vi "ax position control test constant.vi"() -> ()   [LabVIEW 2016]
uses:
  <instrlib>/Dynamixel Motor/Public/Motor Operation/Low Level/Baud Setting.ctl
  <vilib>/myRIO/Instrument Drivers/Onboard IO/DIO/typedefs/DIO Reference.ctl
  <vilib>/myRIO/Common/Instrument Driver Framework/Utilities/typedefs/myRIO Generic Hardware Reference.ctl
  <vilib>/myRIO/Common/Instrument Driver Framework/Utilities/typedefs/Hardware Version Enum.ctl
  <vilib>/myRIO/Common/Instrument Driver Framework/Utilities/typedefs/myRIO v1.0 Reference.ctl
  <vilib>/myRIO/Common/Instrument Driver Framework/Utilities/typedefs/Generic FPGA Reference.ctl
  <vilib>/myRIO/Common/Instrument Driver Framework/myRIO v1.0/DIO/typedefs/DIO Channels List.ctl
  <vilib>/myRIO/Common/Instrument Driver Framework/myRIO v1.0/DIO/typedefs/DIO Channels Enum.ctl
  <vilib>/userdefined/High Color/nirio_resource_hc.ctl
  <vilib>/myRIO/Common/Instrument Driver Framework/Utilities/vis/Is FPGA Ref Available.vi
  <vilib>/myRIO/Common/Instrument Driver Framework/myRIO v1.0/DIO/vis/myRIO v1.1 Open DIO.vi
  <vilib>/myRIO/Instrument Drivers/Onboard IO/DIO/vis/Write.vi
  <vilib>/myRIO/Common/Instrument Driver Framework/Utilities/vis/Validate Channels.vi
  <vilib>/myRIO/Common/Instrument Driver Framework/myRIO v1.0/DIO/vis/myRIO v1.0 Reserve DIO.vi
  <vilib>/myRIO/Common/Instrument Driver Framework/myRIO v1.0/UART/vis/myRIO v1.0 Close UART.vi
  <vilib>/myRIO/Common/Instrument Driver Framework/myRIO v1.0/Resource Manager/vis/myRIO v1.0 Reserve Channel List.vi
  <vilib>/myRIO/Common/Instrument Driver Framework/myRIO v1.0/DIO/vis/myRIO v1.0 Build MUX Configuration DIO.vi
  <vilib>/myRIO/Common/Instrument Driver Framework/myRIO v1.0/Resource Manager/vis/myRIO v1.0 Reserve Channel.vi
  <vilib>/myRIO/Common/Instrument Driver Framework/myRIO v1.0/Resource Manager/vis/myRIO v1.0 Unreserve Channel.vi
  <vilib>/myRIO/Common/Instrument Driver Framework/myRIO v1.0/Resource Manager/vis/myRIO v1.0 Create Configuration List.vi
  <vilib>/myRIO/Common/Instrument Driver Framework/myRIO v1.0/Resource Manager/vis/myRIO v1.0 Build Mutex Name.vi
  <vilib>/Utility/VariantDataType/GetNumericInfo.vi
  <vilib>/Utility/error.llb/Error Cluster From Error Code.vi
  <vilib>/myRIO/Common/Instrument Driver Framework/myRIO v1.0/myRIO v1.1 Open.vi
  <vilib>/myRIO/Common/Instrument Driver Framework/Utilities/vis/IO Manager.vi
  <vilib>/myRIO/Common/Instrument Driver Framework/Utilities/vis/Configuration Manager.vi
  <vilib>/myRIO/Common/Instrument Driver Framework/myRIO v1.0/Resource Manager/vis/myRIO v1.0 Configure IO.vi
  <vilib>/myRIO/Common/Instrument Driver Framework/myRIO v1.0/myRIO v1.0 Close.vi
  <vilib>/myRIO/Common/Instrument Driver Framework/myRIO v1.0/DIO/vis/myRIO v1.0 Write DIO.vi
  <vilib>/myRIO/Common/Instrument Driver Framework/Utilities/vis/FPGA Ref Manager.vi
  <vilib>/myRIO/Common/Instrument Driver Framework/myRIO v1.0/myRIO v1.0 Reset FPGA.vi
  <vilib>/myRIO/Common/Instrument Driver Framework/myRIO v1.0/IRQ/vis/myRIO v1.0 IRQ Info FGV.vi
  <vilib>/myRIO/Common/Instrument Driver Framework/myRIO v1.0/IRQ/vis/myRIO v1.0 Timer IRQ Info FGV.vi
  <vilib>/myRIO/Common/Instrument Driver Framework/myRIO v1.0/IRQ/vis/myRIO v1.0 ISR Agent.vi
  <vilib>/myRIO/Express VI/Onboard Devices/LED/LED Express VI.xnode
  <vilib>/myRIO/Instrument Drivers/Onboard IO/DIO/vis/myRIO DIO Open.xnode
  <instrlib>/Dynamixel Motor/Dynamixel Motor.lvlib
  <vilib>/myRIO/Instrument Drivers/Onboard IO/DIO/DIO.lvlib
  <vilib>/myRIO/Instrument Drivers/Utilities/Utilities.lvlib
panel:
  out "error out 2":errorcluster
  in  "Goal position":dbl=300.0
  out "error out":errorcluster
  in  "LED0":bool
  out "Load/torque %":sgl
  in  "Motor ID (0)":u8=5
  out "Position (deg)":dbl
  in  "정지":bool
  # "Motor 1 Configuration"
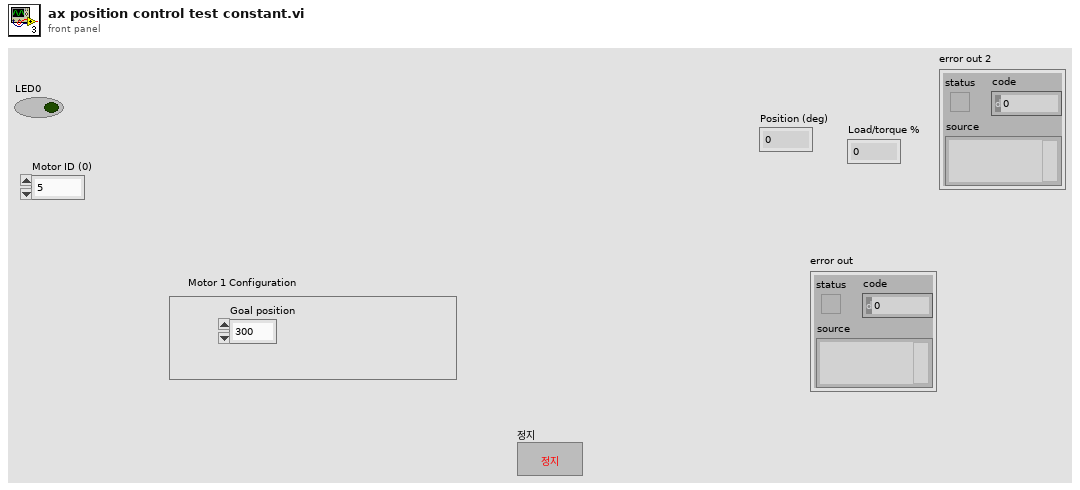
[diagram p1: front panel]
types:
  T1 = typedef "Dynamixel Motor.lvlib/Baud Setting.ctl" = u8
  T2 = typedef "DIO.lvlib/DIO Reference.ctl" = cluster{"myRIO Reference":T3, "DIO Channels List":T7}
  T3 = typedef "myRIO Generic Hardware Reference.ctl" = cluster{"myRIO Model":T4, "myRIO Hardware Reference":T5}
  T4 = typedef "Hardware Version Enum.ctl" = enum16{"Unknown", "myRIO-1900", "myRIO-1950", "roboRIO", "NI ELVIS RIO CM"}
  T5 = typedef "myRIO v1.0 Reference.ctl" = cluster{"Generic FPGA Reference":T6, "Allow multiple opens":bool}
  T6 = typedef "Generic FPGA Reference.ctl" = refnum<k20>
  T7 = typedef "DIO Channels List.ctl" = T8[]
  T8 = typedef "DIO Channels Enum.ctl" = enum16{"Not Connected", "C/DIO0", "C/DIO1", "C/DIO2", "C/DIO3", "C/DIO4", "C/DIO5", "C/DIO6", "C/DIO7", "A/DIO0", "A/DIO1", "A/DIO2", "A/DIO3", "A/DIO4", "A/DIO5", "A/DIO6", "A/DIO7", "A/DIO8", "A/DIO9", "A/DIO10", "A/DIO11", "A/DIO12", "A/DIO13", "A/DIO14", "A/DIO15", "B/DIO0", "B/DIO1", "B/DIO2", "B/DIO3", "B/DIO4", "B/DIO5", "B/DIO6", "B/DIO7", "B/DIO8", "B/DIO9", "B/DIO10", "B/DIO11", "B/DIO12", "B/DIO13", "B/DIO14", "B/DIO15", "LED0", "LED1", "LED2", "LED3", "Button0", "DIO/DIO0", "DIO/DIO1", "DIO/DIO2", "DIO/DIO3", "DIO/DIO4", "DIO/DIO5", "DIO/DIO6", "DIO/DIO7", "DIO/DIO8", "DIO/DIO9", "SPI/CS0", "SPI/CS1", "SPI/CS2", "SPI/CS3", "LED RADIO (Green)", "LED RADIO (Red)", "LED COMM (Green)", "LED COMM (Red)", "LED MODE (Green)", "LED MODE (Red)"}
  T9 = typedef "nirio_resource_hc.ctl" = tag
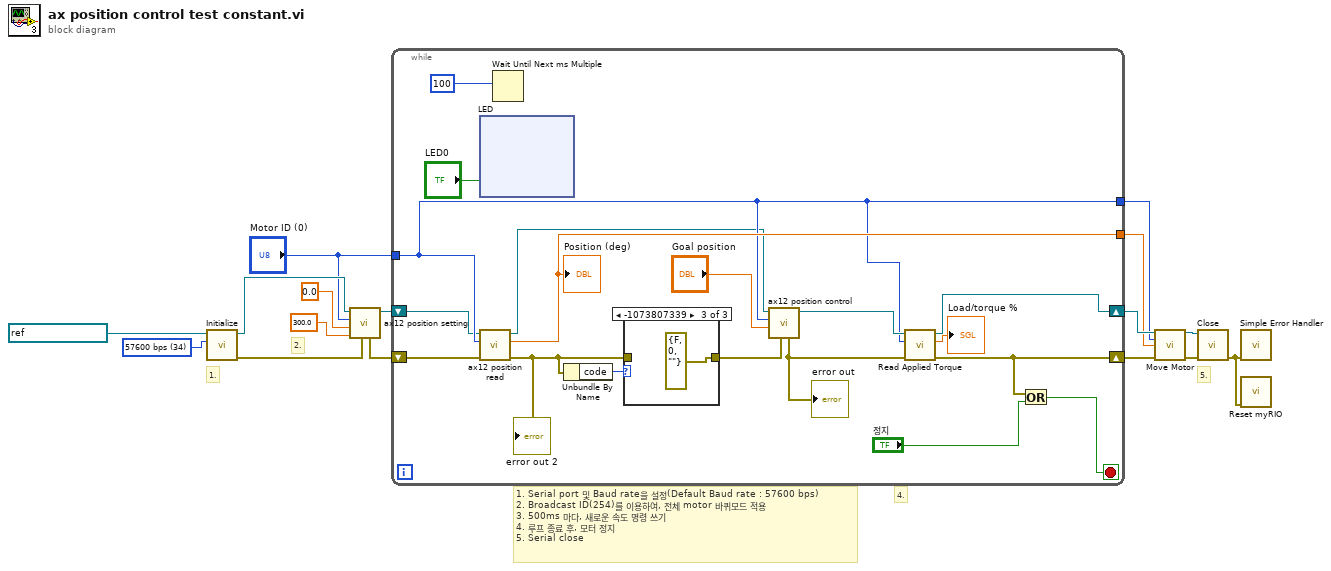
[diagram p0: block diagram]
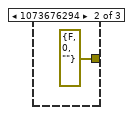
[diagram p3: hidden frame]
diagram:
  w16 = T1 34 items=["1,000,000 bps"=1, "500,000 bps"=3, "400,000 bps"=4, "250,000 bps"=7, "200,000 bps"=9, "115200 bps"=16, "57600 bps"=34, "19200 bps"=103, "9600 bps"=207] ("Baud rate (57600 bps)")
  # "5."
  # "1. Serial port 및 Baud rate을 설정(Default Baud rate : 57600 bps)\n2. Broadcast ID(254)를 이용하여, 전체 motor 바퀴모드 적용\n3. 500ms 마다, 새로운 속도 명령 쓰기\n4. 루프 종료 후, 모터 정지\n5. Serial close"
  # "2."
  # "4."
  # "1."
  n1 = call <instrlib>:"Initialize.vi"("Baud rate (57600 bps)"=w16, "VISA resource name"=refnum<visa-resource-name> "ASRL3::INSTR") -> ("error out"=w8:errorcluster, "VISA resource name out"=w6:refnum<visa-resource-name>)  [unwired: 8 in]
  n2 = call "ax12 position setting.vi"("error in (no error)"=w8, "Counter-Clockwise Angle Limit (300 deg)"=300.0, "Clockwise Angle Limit (0 deg)"=0.0, "Motor ID (0)"="Motor ID (0)", "VISA resource name"=w6) -> ("VISA resource name out"=w5:refnum<visa-resource-name>, "error out"=w7:errorcluster)  [unwired: 5 in]
  n3 = while {
    shift-right: [w34] -> w14
    shift-left: w5 -> [w26]
    shift-right: [w21] -> w13
    shift-left: w7 -> [w29]
    tunnel: "Motor ID (0)" -> [w27]
    tunnel: [w27] -> w11
    tunnel: [w28] -> w9
    stop <- w19 stop-if-true
    n4 = xnode "LED"("LED0"="LED0") -> ()  [unwired: 1 in, 1 out]
    n5 = call "ax12 position read.vi"("error in (no error)"=w29, "Motor ID (0)"=w27, "VISA resource name"=w26) -> ("error out"=w22:errorcluster, "Position (deg)"=w28:dbl, "VISA resource name out"=w25:refnum<visa-resource-name>)  [unwired: 6 in]
    "Position (deg)" <- w28
    "error out 2" <- w22
    n6 = Wait Until Next ms Multiple(millisecond multiple=u32 100 ("대기 시간 (ms)")) -> ()  [unwired: 1 out]
    n7 = Unbundle By Name(w22) -> ("code"=w18:i32)
    n8 = case shown="-1073807339" w18 {
      tunnel: [w35 errorcluster {"status"=FALSE, "code"=0, "source"=""} ("에러 출력") errorcluster {"status"=FALSE, "code"=0, "source"=""} ("에러 출력")] -> w31
      tunnel: w22 -> [w35 _ _]
      frame 0, Default {
      }
      frame 1073676294 {
      }
      frame -1073807339 {
      }
    }
    n9 = call "ax12 position control.vi"("error in (no error)"=w31, "Goal Position (180 deg)"="Goal position", "Motor ID (0)"=w27, "VISA resource name"=w25) -> ("VISA resource name out"=w32:refnum<visa-resource-name>, "error out"=w24:errorcluster)  [unwired: 6 in]
    "error out" <- w24
    n10 = call <instrlib>:"Read Applied Torque.vi"("error in (no error)"=w24, "Motor ID (0)"=w27, "VISA resource name"=w32) -> ("error out"=w21:errorcluster, "Load/torque %"=→"Load/torque %":sgl, "VISA resource name out"=w34:refnum<visa-resource-name>)  [unwired: 6 in]
    n11 = Or(x=w21, y="정지") -> (x .or. y?=w19:bool)
  }
  n12 = call <instrlib>:"Move Motor.vi"("VISA resource name"=w14, "Motor ID (0)"=w11, "Goal Position (180 deg)"=w9, "error in (no error)"=w13) -> ("VISA resource name out"=w12:refnum<visa-resource-name>, "error out"=w15:errorcluster)  [unwired: 10 in]
  n13 = call <instrlib>:"Close.vi"("error in (no error)"=w15, "VISA resource name"=w12) -> ("error out"=w1:errorcluster)  [unwired: 9 in]
  n14 = call <vilib>:"Simple Error Handler.vi"("error in (no error)"=w1) -> ()  [unwired: 4 in, 5 out]
  n15 = call <vilib>:"Reset myRIO.vi"("error in (no error)"=w1) -> ()  [unwired: 10 in, 1 out]
